vi "运维调试_CODCr.vi"() -> ()   [LabVIEW 2016, in "CODCr库.lvlib"]
uses:
  <vilib>/Utility/miscctls.llb/LVPointTypeDef.ctl
  <vilib>/ptbypt/NI_PtbyPt.lvlib
  <vilib>/Utility/config.llb/NI_LVConfig.lvlib
panel:
  out "数据时间":timestamp format="%<%Y/%m/%d %H:%M:%S>T"
  in  "质控参数":bool
  in  "仪器参数":bool
  in  "MB通信方式选择":enum16{"串口", "TCP"}(ring)
  in  "释放串口":bool
  in  "打开串口":bool
  in  "加标回收测试":bool
  in  "平行样测试":bool
  in  "定时启动":bool
  out "COM口":string
  in  "空白测试":bool
  in  "隐藏按钮":bool
  in  "写入消解温度时长":bool
  in  "保存KB值":bool
  in  "标样核查":bool
  out "启动时间":timestamp format="%<%Y/%m/%d %H:%M:%S>T"
  out "主循环次数":i32
  out "status":bool
  out "启动测量模式":T1(ring)
  out "曲线截距B":sgl format="%#_10g"
  out "曲线斜率K":sgl format="%#_10g"
  out "量程上限":sgl
  out "量程下限":sgl
  out "消解时长":u16
  out "消解温度":u16
  out "测量精度":u16
  out "测量结果":sgl
  out "标样参考值":sgl
  out "量程":u16
  out "工作状态":T1(ring)
  out "仪器时间":timestamp format="%<%X\n%x>T"
  out "关键参数区":T2
  out "状态告警区":T3 {"告警代码" items=["无告警", "缺试剂告警", "缺水样告警", "缺蒸馏水告警", "缺标液告警", "仪表漏液告警", "标定异常告警", "超量程告警", "加热异常", "低试剂预警", "超上限告警", "超下限告警", "仪表内部其他异常", "滴定异常告警", "电极异常告警", "量程切换告警", "参数设置告警", "PH电极电位异常", "电导率电极异常", "浊度光度异常", "溶解氧电极异常", "溶解氧光强异常", "温度异常告警", "PH异常告警", "溶解氧异常告警", "电导率异常告警", "浊度异常告警", "叶绿素异常告警", "藻密度异常告警", "蓝绿藻异常告警", "ORP异常告警", "氨氮异常告警", "清洁刷异常告警", "SD卡异常告警", "蓝牙异常告警", "Wifi异常告警", "流程异常告警"]; "故障代码" items=["无故障", "电机故障", "温度故障", "通讯故障", "滴定故障"]}
  out "测量数据区":T4 {"单位" items=["ug/L", "mg/L", "ppm", "mg/m3", "cm", "ppb", "ug/m3", "%", "nmol/mol", "umol/mol", "MPN/L", "MPN/100ml", "ng/m3", "NTU", "无量纲", "ms/cm", "us/cm", "℃", "mV", "万个/L"]}
  out "系统时间":timestamp format="%<%Y/%m/%d %H:%M:%S>T"
  in  "停止":bool
  in  "校时":bool
  in  "标样校准":bool
  in  "空白校准":bool
  in  "零点核查":bool
  in  "跨度核查":bool
  in  "水样测试":bool
  in  "返回":bool
  in  "设置":bool
  # "mg/L"
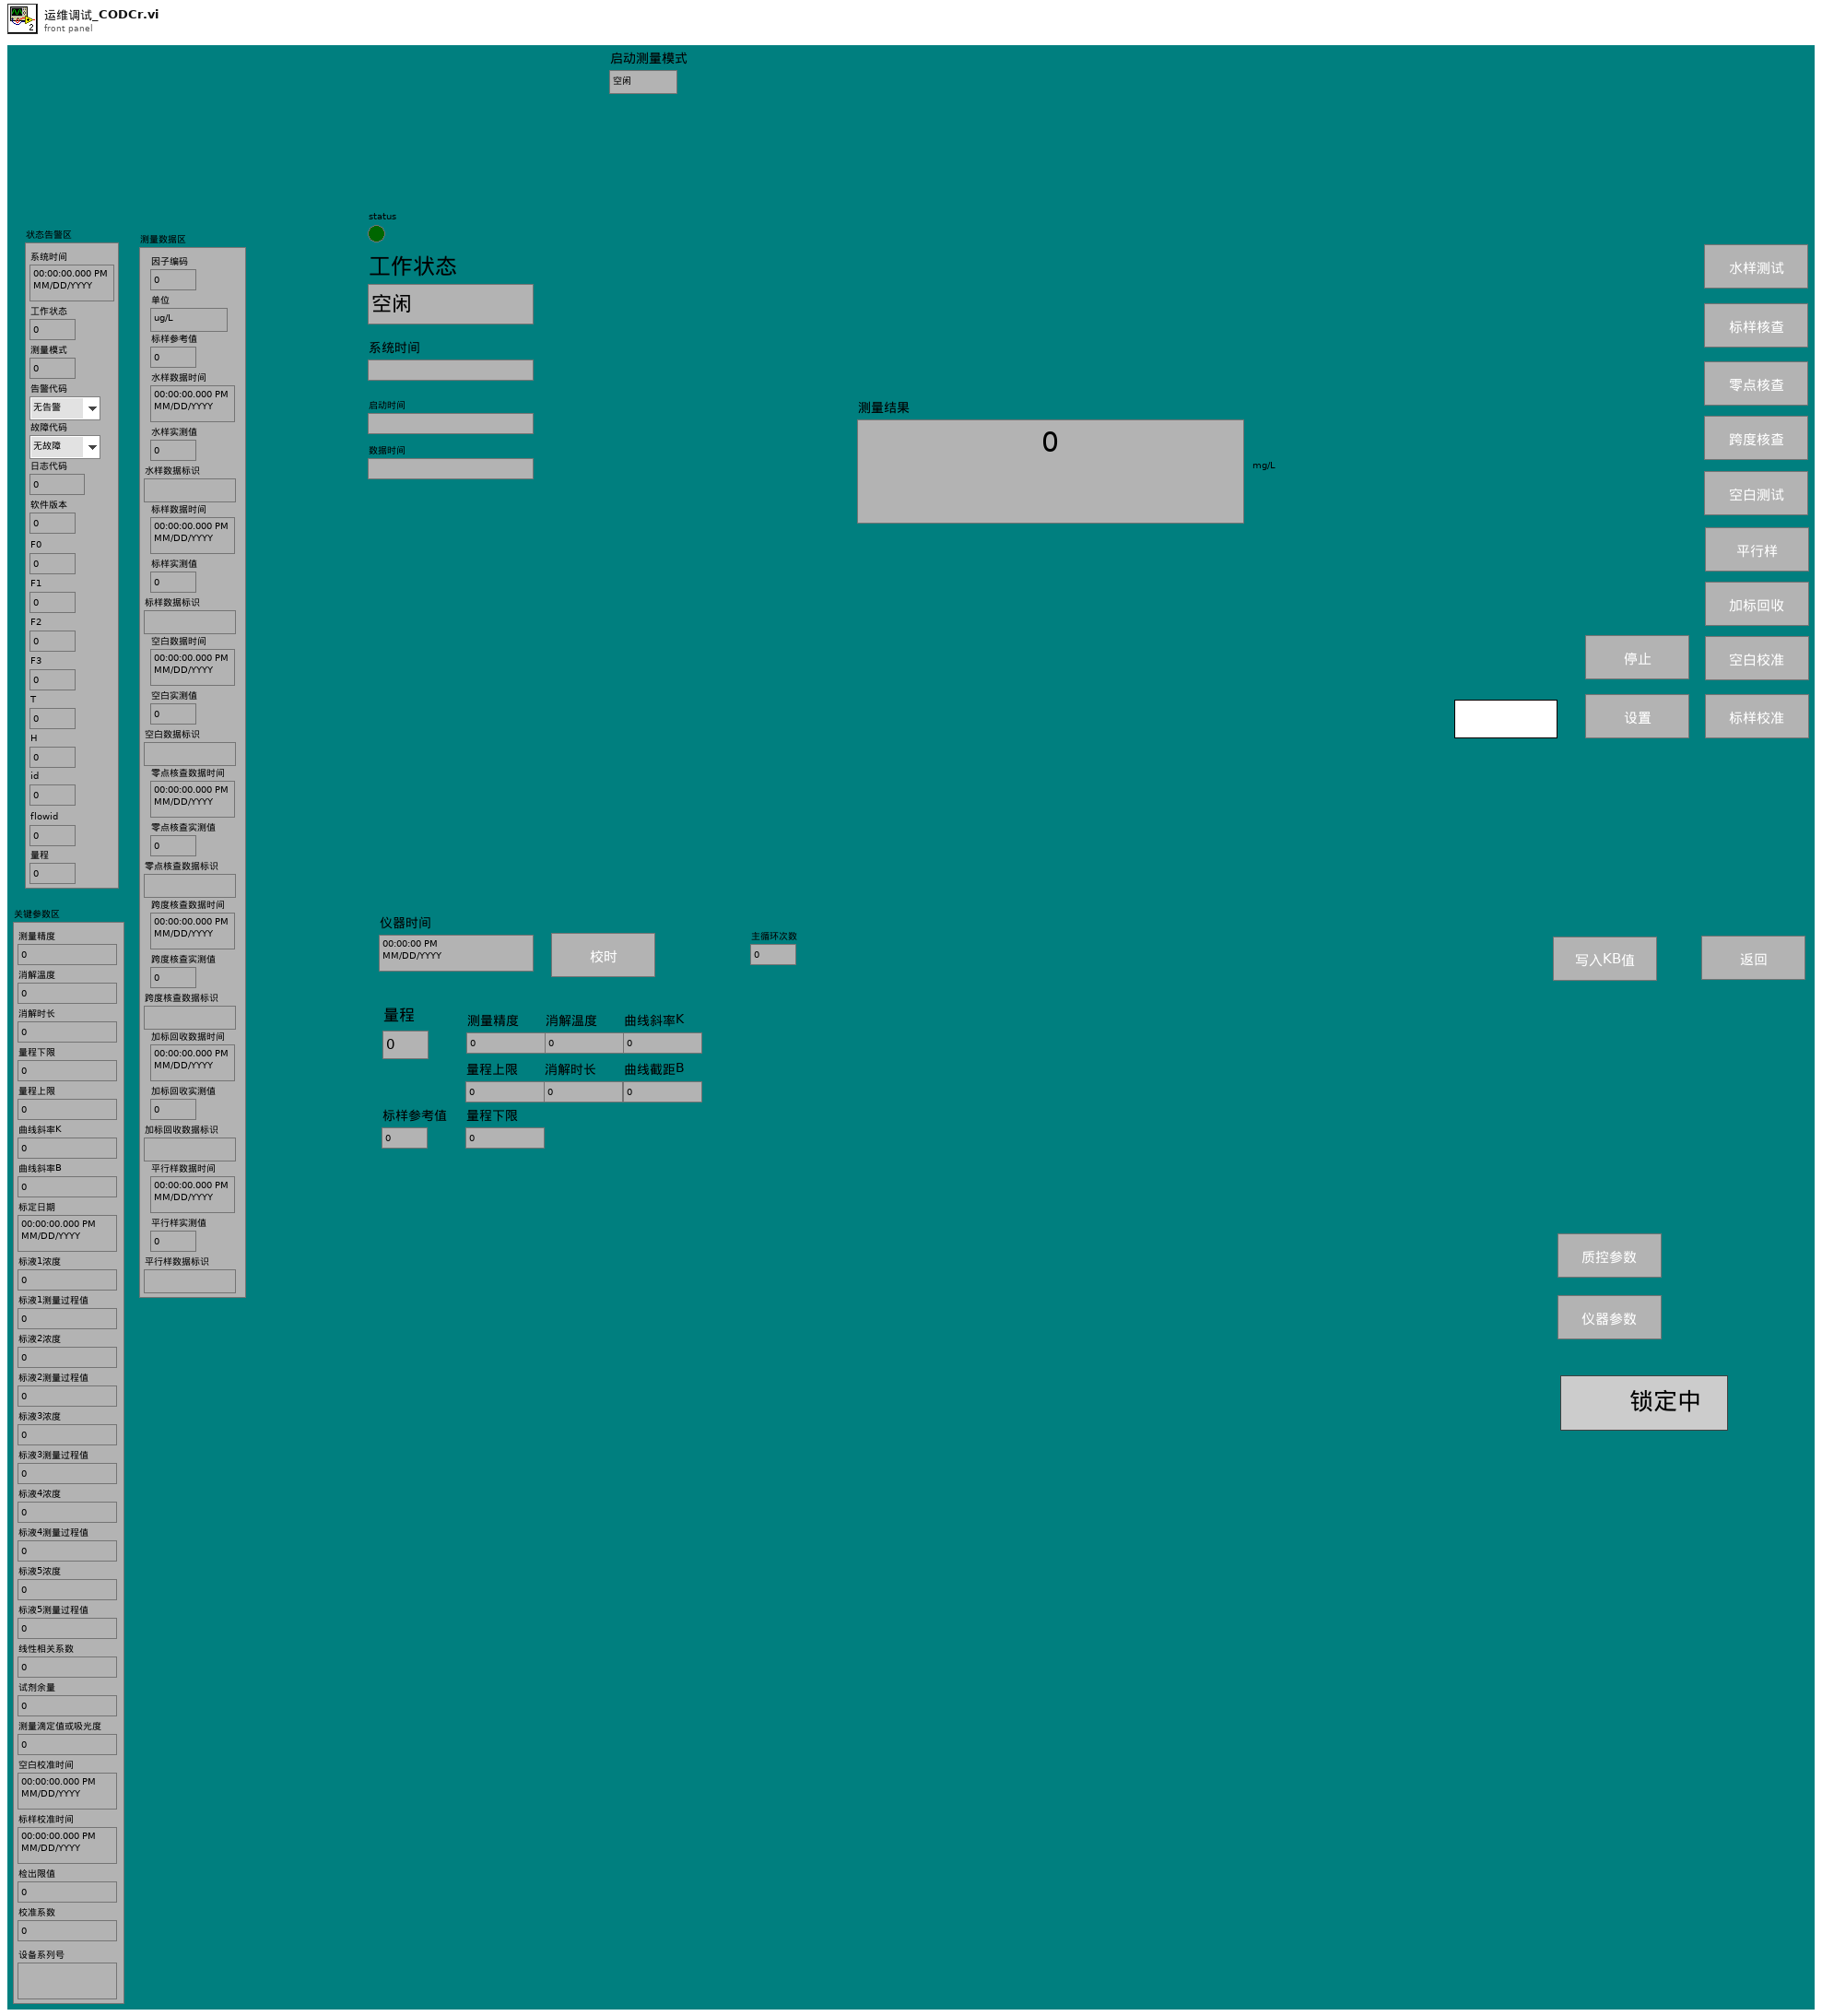
[diagram p1: front panel]
types:
  T1 = enum16{"空闲", "水样测试", "标样核查", "零点核查", "跨度核查", "空白测试", "平行样测试", "加标回收", "空白校准", "标样校准", "初始化（清洗）"}
  T2 = cluster{"测量精度":u16, "消解温度":u16, "消解时长":u16, "量程下限":sgl, "量程上限":sgl, "曲线斜率K":sgl, "曲线斜率B":sgl, "标定日期":timestamp, "标液1浓度":sgl, "标液1测量过程值":sgl, "标液2浓度":sgl, "标液2测量过程值":sgl, "标液3浓度":sgl, "标液3测量过程值":sgl, "标液4浓度":sgl, "标液4测量过程值":sgl, "标液5浓度":sgl, "标液5测量过程值":sgl, "线性相关系数":sgl, "试剂余量":u32, "测量滴定值或吸光度":sgl, "空白校准时间":timestamp, "标样校准时间":timestamp, "检出限值":sgl, "校准系数":sgl, "设备系列号":string}
  T3 = cluster{"系统时间":timestamp, "工作状态":u16, "测量模式":u16, "告警代码":u16, "故障代码":u16, "日志代码":u16, "软件版本":u16, "F0":sgl, "F1":sgl, "F2":sgl, "F3":sgl, "T":sgl, "H":sgl, "id":u16, "flowid":u16, "量程":u16}
  T4 = cluster{"因子编码":u32, "单位":u16, "标样参考值":sgl, "水样数据时间":timestamp, "水样实测值":sgl, "水样数据标识":string, "标样数据时间":timestamp, "标样实测值":sgl, "标样数据标识":string, "空白数据时间":timestamp, "空白实测值":sgl, "空白数据标识":string, "零点核查数据时间":timestamp, "零点核查实测值":sgl, "零点核查数据标识":string, "跨度核查数据时间":timestamp, "跨度核查实测值":sgl, "跨度核查数据标识":string, "加标回收数据时间":timestamp, "加标回收实测值":sgl, "加标回收数据标识":string, "平行样数据时间":timestamp, "平行样实测值":sgl, "平行样数据标识":string}
  T5 = cluster{"命令":string, "测量模式":enum16{"水样测量", "标样核查", "零点核查", "跨度核查", "空白测试", "加标回收", "平行样", "校零", "校标"}, "CODCr量程切换":enum32{"H", "L", "AUTO"}}
  T6 = typedef "LVPointTypeDef.ctl" = cluster{"Horizontal":i16, "Vertical":i16}
  T7 = typedef "NI_LVConfig.lvlib/Config Data RefNum.ctl" = refnum<k1>
  T8 = cluster{"运行模式":enum16{"维护模式", "常规模式", "应急模式", "质控模式"}}
  T9 = cluster{"时间标识":timestamp, "监测值":sgl, "单位":u16, "数据标识":string, "因子编码":u32, "标样参考值":sgl, "F0":sgl, "F1":sgl, "F2":sgl, "F3":sgl, "温度":sgl, "湿度":sgl, "量程标识":string, "LastTime":timestamp}
  T10 = cluster{"时间标识":timestamp, "设备":string, "日志信息":string}
  T11 = cluster{"时间标识":timestamp, "参数":string, "日志信息":string, "流程参数":string}
  T12 = cluster{"时间标识":timestamp, "设备":string, "日志信息":string, "流程参数":string}
  T13 = enum16{"水样测量", "标样核查", "零点核查", "跨度核查", "空白测试", "加标回收", "平行样", "校零", "校标"}
  T14 = cluster{"控制命令":enum16{"启动测量", "标样核查", "零点核查", "跨度核查", "空白测试", "平行样测试", "加标回收", "空白校准", "标样校准", "初始化（清洗）", "停止测试", "仪器重启", "校时", "模式设置", "测量间隔设置"}, "周期设置类型":enum16{"定点启动", "间隔启动"}, "定时功能启用":bool, "定时间隔":dbl, "24H周期设置":bool[], "零点核查时间":u16, "跨度核查时间":u16, "质控频次":enum16{"关闭", "每天", "星期一", "星期二", "星期三", "星期四", "星期五", "星期六", "星期日"}}
  T15 = cluster{"测量量程":dbl, "测量精度":dbl, "测量间隔":dbl, "消解温度":dbl, "消解时长":dbl, "空白校准时间":timestamp, "曲线截距":dbl, "曲线斜率":dbl, "测量检出限":dbl, "测量信号值":dbl, "线性相关系数":dbl, "二次多项式系数":dbl, "标样校准时间":timestamp, "稀释倍数":dbl, "三项式系数":dbl, "空白标定系数":dbl, "量程系数":dbl, "F0/ORPA":dbl, "F1/ORPB":dbl, "F2/ORPK":dbl, "F3":dbl, "F4":dbl, "F5":dbl, "F6":dbl, "F7":dbl, "X0/滴定数":dbl, "量程":dbl}
  T16 = cluster{"控制命令":enum16{"启动测量", "标样核查", "零点核查", "跨度核查", "空白测试", "平行样测试", "加标回收", "空白校准", "标样校准", "初始化（清洗）", "停止测试", "仪器重启", "校时", "模式设置", "测量间隔设置"}, "周期设置类型":enum16{"定点启动", "间隔启动"}, "定时功能启用":bool, "定时间隔":dbl, "24H周期设置":bool[], "空白核查时间":u16, "跨度核查时间":u16, "质控频次":enum16{"关闭", "每天", "星期一", "星期二", "星期三", "星期四", "星期五", "星期六", "星期日"}}
  T17 = cluster{"确定":bool, "测量量程":dbl, "测量精度":dbl, "测量间隔":dbl, "消解温度":dbl, "消解时长":dbl, "空白校准时间":timestamp, "曲线截距":dbl, "曲线斜率":dbl, "测量检出限":dbl, "测量信号值":dbl, "线性相关系数":dbl, "二次多项式系数":dbl, "标样校准时间":timestamp, "稀释倍数":dbl, "三项式系数":dbl, "空白标定系数":dbl, "量程系数":dbl, "F0/ORPA":dbl, "F1/ORPB":dbl, "F2/ORPK":dbl, "F3":dbl, "F4":dbl, "F5":dbl, "F6":dbl, "F7":dbl, "X0/滴定数":dbl, "量程":dbl}
  T18 = cluster{"跨度值":dbl, "零点标准液浓度":dbl, "跨度标准液浓度":dbl, "标准液标准浓度":dbl}
  T19 = cluster{"确定":bool, "跨度值":dbl, "零点标准液浓度":dbl, "跨度标准液浓度":dbl, "标准液标准浓度":dbl}
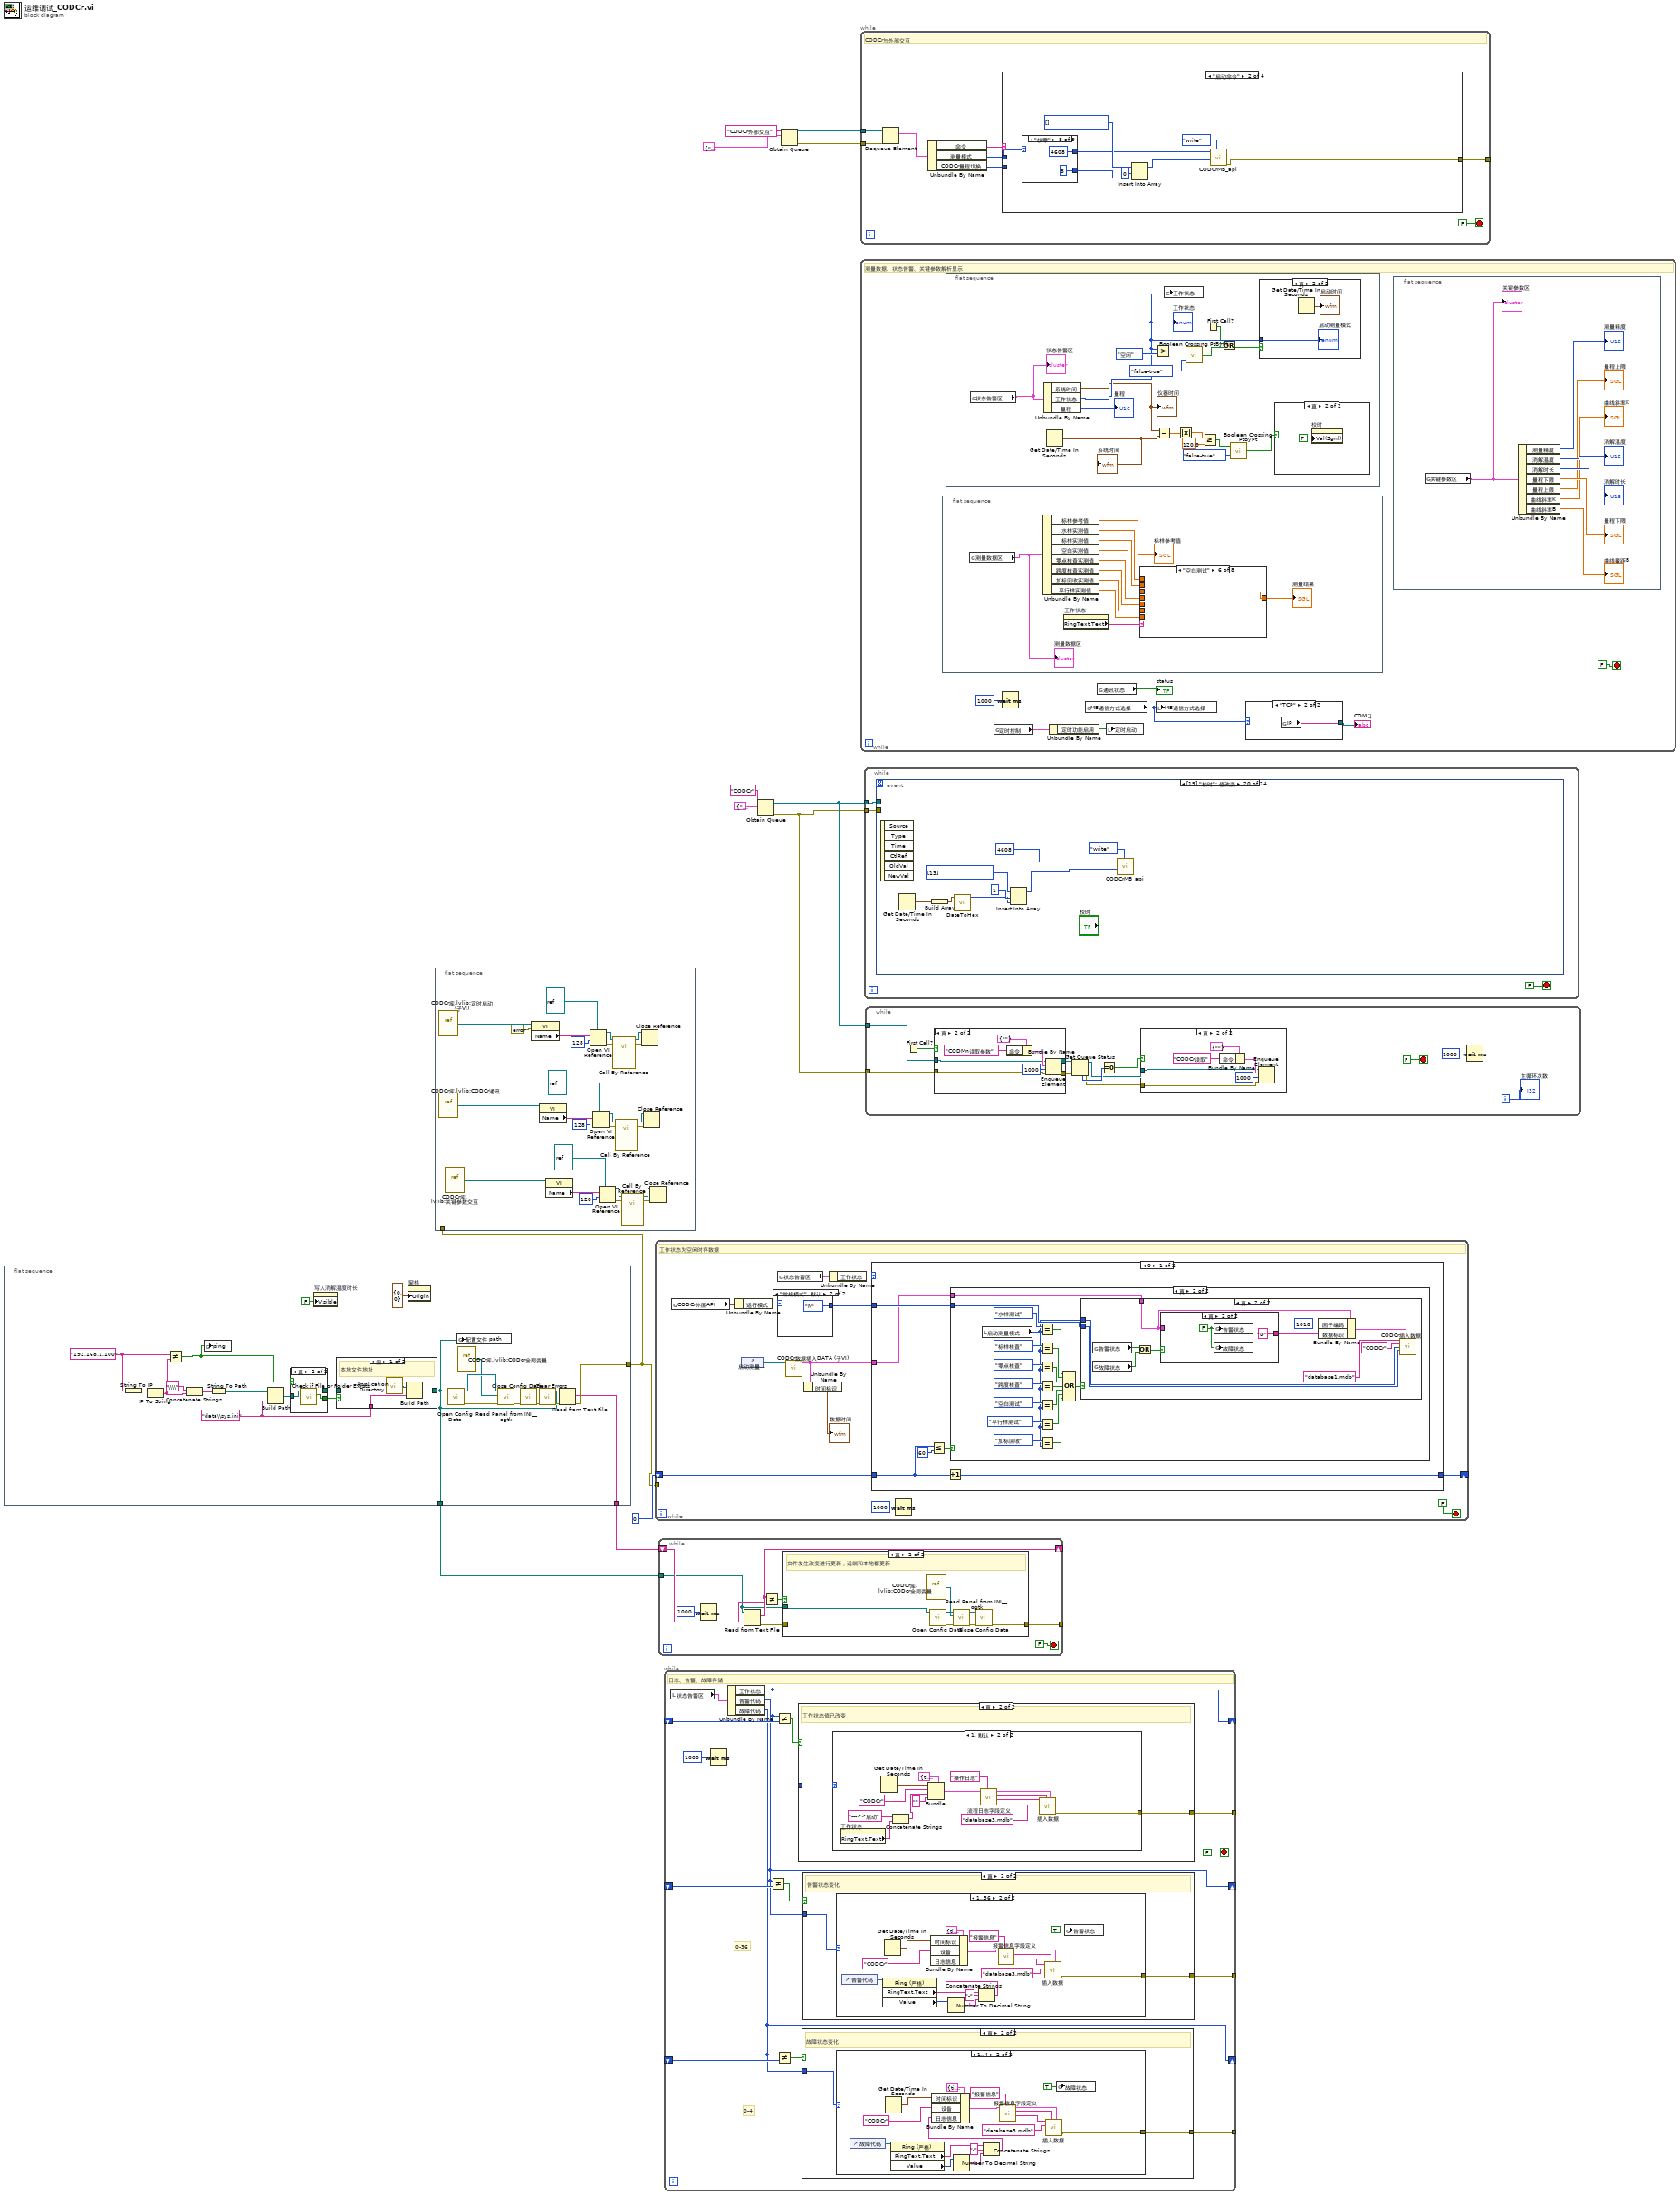
[diagram p0: block diagram]
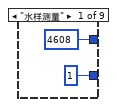
[diagram p6: hidden frame]
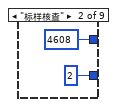
[diagram p7: hidden frame]
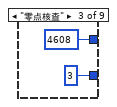
[diagram p8: hidden frame]
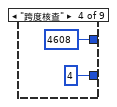
[diagram p9: hidden frame]
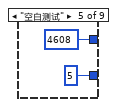
[diagram p10: hidden frame]
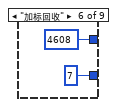
[diagram p11: hidden frame]
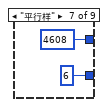
[diagram p12: hidden frame]
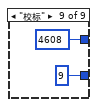
[diagram p13: hidden frame]
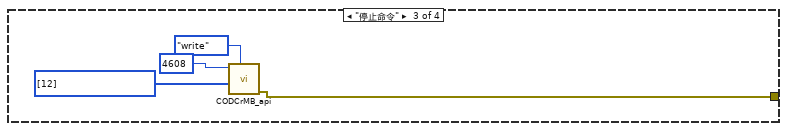
[diagram p14: hidden frame]
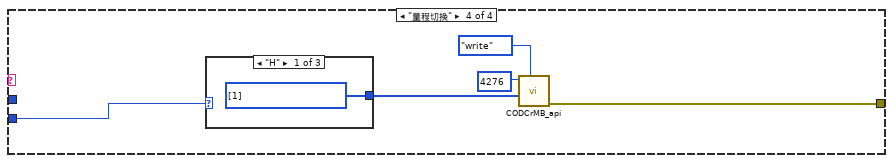
[diagram p15: hidden frame]
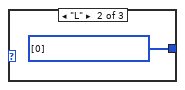
[diagram p16: hidden frame]
diagram:
  n1 = flat-sequence {
    tunnel: [w15] -> w1
    tunnel: [w14] -> w3
    tunnel: [w13] -> w2
    frame #0 {
      w33 = "data\\sys.ini" ("名称或相对路径")
      w18 = "192.168.1.100" ("名称")
      n2 = String To IP(1:w18) -> (0:w25:u32)
      n3 = IP To String(2:w25) -> (0:w22:string)  [unwired: 1 in]
      n4 = Not Equal?(x=w18, y=w22) -> (x != y?=w32:bool)
      n5 = Concatenate Strings("\\\\" ("字符串"), w22) -> (w23:string)
      n6 = global write "CODcr全局变量.vi" "ping"(w32) -> ()
      n7 = String To Path(string=w23) -> (path=w17:path)
      n8 = Build Path(base path=w17, name or relative path=w33) -> (appended path=w21:path)
      n9 = case shown="真" w32 {
        tunnel: w21 -> [w36 w40]
        tunnel: [w36 w39] -> w20
        tunnel: [FALSE w38] -> w19
        frame False {
        }
        frame True {
          n10 = call <vilib>:"Check if File or Folder Exists.vi"("path"=w40) -> ("file or folder exists?"=w38:bool, "dup path"=w39:path)  [unwired: 8 in, 1 out]
        }
      }
      n11 = property on="写入消解温度时长" class="Bool"("Visible"=FALSE ("可见")) -> ()  [unwired: 2 in, 2 out]
      n12 = case shown="假" w19 {
        tunnel: w20 -> [_ w44]
        tunnel: [w42 w44] -> w13
        tunnel: w33 -> [w41 _]
        frame False {
          # "本地文件地址"
          n13 = call <vilib>:"Application Directory.vi"() -> ("Application Directory"=w43:path)
          n14 = Build Path(base path=w43, name or relative path=w41) -> (appended path=w42:path)
        }
        frame True {
          # "网络共享地址"
        }
      }
      n15 = property on="窗格" class="Pane"("Origin"=T6 {"Horizontal"=0, "Vertical"=0} ("原点")) -> ()  [unwired: 2 in, 2 out]
      n16 = call <vilib>:"Open Config Data.vi"("configuration file path"=w13) -> ("error out"=w29:errorcluster, "refnum"=w28:T7)  [unwired: 8 in, 1 out]
      n17 = global write "CODcr全局变量.vi" "配置文件 path"(w13) -> ()
      n18 = vi-ref "CODCr库.lvlib:CODcr全局变量.vi"() -> (w16:refnum<vi>)
      n19 = call <userlib>:"Read Panel from INI__ogtk.vi"("error in (no error)"=w29, "VI ref"=w16, "refnum"=w28) -> ("error out"=w27:errorcluster, "refnum out"=w26:T7)  [unwired: 7 in]
      n20 = call <vilib>:"Close Config Data.vi"("error in (no error)"=w27, "refnum"=w26) -> ("error out"=w30:errorcluster)  [unwired: 8 in, 1 out]
      n21 = call <vilib>:"Clear Errors.vi"("error in (no error)"=w30) -> ("error out"=w31:errorcluster)  [unwired: 5 in, 1 out]
      n22 = Read from Text File(file (use dialog)=w13, error in=w31) -> (text=w14:string, error out=w15:errorcluster)  [unwired: 2 in, 2 out]
    }
  }
  n23 = flat-sequence {
    tunnel: w1 -> [_]
    frame #0 {
      n24 = vi-ref "CODCr库.lvlib:定时启动 (子VI).vi"() -> (w53:refnum<vi>)
      n25 = vi-ref "CODCr库.lvlib:CODCr通讯.vi"() -> (w62:refnum<vi>)
      n26 = vi-ref "CODCr库.lvlib:关键参数交互.vi"() -> (w52:refnum<vi>)
      n27 = property class="VI"(reference=w53, error in=errorcluster {"status"=FALSE, "code"=0, "source"=""} ("错误输出")) -> ("Name"=w54:string)  [unwired: 2 out]
      n28 = property class="VI"(reference=w62) -> ("Name"=w63:string)  [unwired: 1 in, 2 out]
      n29 = property class="VI"(reference=w52) -> ("Name"=w51:string)  [unwired: 1 in, 2 out]
      n30 = Open VI Reference(type specifier VI Refnum (for type only)=refnum<vi> refnum, vi path=w54, options=128 ("选项")) -> (vi reference=w56:refnum<vi>, error out=w58:errorcluster)  [unwired: 3 in]
      n31 = Open VI Reference(type specifier VI Refnum (for type only)=refnum<vi> refnum, vi path=w63, options=128 ("选项")) -> (vi reference=w65:refnum<vi>, error out=w67:errorcluster)  [unwired: 3 in]
      n32 = Open VI Reference(type specifier VI Refnum (for type only)=refnum<vi> refnum, vi path=w51, options=128 ("选项")) -> (vi reference=w49:refnum<vi>, error out=w47:errorcluster)  [unwired: 3 in]
      n33 = call-by-ref "?"(reference=w56, error in=w58) -> (reference out=w60:refnum<vi>, error out=w59:errorcluster)  [unwired: 12 in]
      n34 = call-by-ref "?"(reference=w65, error in=w67) -> (reference out=w69:refnum<vi>, error out=w68:errorcluster)  [unwired: 12 in]
      n35 = call-by-ref "?"(reference=w49, error in=w47) -> (reference out=w45:refnum<vi>, error out=w46:errorcluster)  [unwired: 12 in]
      n36 = Close Reference(reference=w60, error in (no error)=w59) -> ()  [unwired: 1 out]
      n37 = Close Reference(reference=w69, error in (no error)=w68) -> ()  [unwired: 1 out]
      n38 = Close Reference(reference=w45, error in (no error)=w46) -> ()  [unwired: 1 out]
    }
  }
  n39 = while "While循环" {
    tunnel: w1 -> [_]
    shift-right: [w73] -> _
    shift-left: 0 -> [w74]
    stop <- FALSE stop-if-true
    # "工作状态为空闲时存数据"
    n40 = global read "CODCr外部API.vi" "CODCr外围API"() -> (w77:T8)
    n41 = Unbundle By Name(w77) -> ("运行模式"=w76:enum16{"维护模式", "常规模式", "应急模式", "质控模式"})
    n42 = control-ref of="启动测量模式"() -> (w72:refnum<vi>)
    n43 = global read "CODcr全局变量.vi" "状态告警区"() -> (w75:T3)
    n44 = case shown="\"常规模式\", 默认" w76 {
      tunnel: [enum16{"N", "M"}."M" ("数据类型") enum16{"N", "M"}."N" ("数据类型")] -> w78
      frame "维护模式" {
      }
      frame "常规模式", Default {
      }
    }
    n45 = call "CODCr数据插入DATA (子VI).vi"("Enum输入"=w72) -> ("data"=w71:T9)  [unwired: 10 in]
    n46 = Unbundle By Name(w71) -> ("时间标识"=→"数据时间":timestamp)
    n47 = Unbundle By Name(w75) -> ("工作状态"=w79:u16)
    n48 = case shown="0" w79 {
      tunnel: w78 -> [w89 _]
      tunnel: w74 -> [w87 _]
      tunnel: [w88 _] -> w73
      tunnel: w71 -> [w84 _]
      frame 0 {
        n49 = Less Or Equal?(x=w87, y=60) -> (x <= y?=w85:bool)
        n50 = Increment(x=w87) -> (x+1=w88:i32)
        n51 = case shown="真" w85 {
          tunnel: w89 -> [_ w107]
          tunnel: w84 -> [_ w90]
          frame False {
          }
          frame True {
            n52 = local read "启动测量模式"() -> (w99:T1)
            n53 = Equal?(x=T1."水样测试" ("启动测量模式"), y=w99) -> (x = y?=w98:bool)
            n54 = Equal?(x=T1."标样核查" ("启动测量模式"), y=w99) -> (x = y?=w97:bool)
            n55 = Equal?(x=T1."零点核查" ("启动测量模式"), y=w99) -> (x = y?=w96:bool)
            n56 = Equal?(x=T1."跨度核查" ("启动测量模式"), y=w99) -> (x = y?=w95:bool)
            n57 = Equal?(x=T1."空白测试" ("启动测量模式"), y=w99) -> (x = y?=w94:bool)
            n58 = Equal?(x=T1."平行样测试" ("启动测量模式"), y=w99) -> (x = y?=w93:bool)
            n59 = Equal?(x=T1."加标回收" ("启动测量模式"), y=w99) -> (x = y?=w92:bool)
            n60 = Compound Arithmetic op=OR(w98, w97, w96, w95, w94, w93, w92) -> (w91:bool)
            n61 = case shown="真" w91 {
              tunnel: w99 -> [_ w115]
              tunnel: w107 -> [_ w114]
              tunnel: w90 -> [_ w108]
              frame False {
              }
              frame True {
                n62 = global read "CODcr全局变量.vi" "告警状态"() -> (w112:bool)
                n63 = global read "CODcr全局变量.vi" "故障状态"() -> (w111:bool)
                n64 = Or(x=w112, y=w111) -> (x .or. y?=w110:bool)
                n65 = case shown="真" w110 {
                  tunnel: w108 -> [w120 _]
                  tunnel: [w119 "D" ("table")] -> w109
                  frame False {
                    n66 = Unbundle By Name(w120) -> ("数据标识"=w119:string)
                  }
                  frame True {
                    w121 = FALSE ("告警状态")
                    n67 = global write "CODcr全局变量.vi" "告警状态"(w121) -> ()
                    n68 = global write "CODcr全局变量.vi" "故障状态"(w121) -> ()
                  }
                }
                n69 = Bundle By Name(cluster=w108, "因子编码"=u32 1018, "数据标识"=w109) -> (w118:T9)
                n70 = call "CODCr插入数据.vi"("database"="database1.mdb", "data"=w118, "table"="CODCr", "测量模式"=w115, "数据类型"=w114) -> ()  [unwired: 10 in, 1 out]
              }
            }
          }
        }
      }
      frame 1, Default {
      }
    }
    n71 = Wait (ms)(milliseconds to wait=u32 1000 ("等待时间（毫秒）")) -> ()  [unwired: 1 out]
  }
  n72 = while {
    tunnel: [w129] -> _
    shift-right: [w127] -> _
    shift-left: w3 -> [w126]
    tunnel: w2 -> [w123]
    stop <- FALSE stop-if-true
    n73 = Wait (ms)(milliseconds to wait=u32 1000 ("等待时间（毫秒）")) -> ()  [unwired: 1 out]
    n74 = Read from Text File(file (use dialog)=w123) -> (text=w127:string, error out=w124:errorcluster)  [unwired: 3 in, 2 out]
    n75 = Not Equal?(x=w127, y=w126) -> (x != y?=w125:bool)
    n76 = case shown="真" w125 {
      tunnel: [w131 w138] -> w129
      tunnel: w123 -> [_ w132]
      tunnel: w124 -> [w131 _]
      frame False {
      }
      frame True {
        # "文件发生改变进行更新，远端和本地都更新"
        n77 = vi-ref "CODCr库.lvlib:CODcr全局变量.vi"() -> (w133:refnum<vi>)
        n78 = call <vilib>:"Open Config Data.vi"("configuration file path"=w132) -> ("error out"=w137:errorcluster, "refnum"=w136:T7)  [unwired: 8 in, 1 out]
        n79 = call <userlib>:"Read Panel from INI__ogtk.vi"("error in (no error)"=w137, "VI ref"=w133, "refnum"=w136) -> ("error out"=w135:errorcluster, "refnum out"=w134:T7)  [unwired: 7 in]
        n80 = call <vilib>:"Close Config Data.vi"("error in (no error)"=w135, "refnum"=w134) -> ("error out"=w138:errorcluster)  [unwired: 8 in, 1 out]
      }
    }
  }
  n81 = while {
    shift-right: [w149] -> _
    shift-left: _ -> [w151]
    tunnel: [w148] -> _
    shift-right: [w145] -> _
    shift-left: _ -> [w146]
    shift-right: [w141] -> _
    shift-left: _ -> [w143]
    tunnel: [w142] -> _
    tunnel: [w140] -> _
    stop <- FALSE stop-if-true
    # "0-4"
    # "0-36"
    # "日志、告警、故障存储"
    n82 = local read "状态告警区"() -> (w139:T3)
    n83 = Wait (ms)(milliseconds to wait=u32 1000 ("等待时间（毫秒）")) -> ()  [unwired: 1 out]
    n84 = Unbundle By Name(w139) -> ("工作状态"=w149:u16, "告警代码"=w145:u16, "故障代码"=w141:u16)
    n85 = Not Equal?(x=w145, y=w146) -> (x != y?=w147:bool)
    n86 = Not Equal?(x=w149, y=w151) -> (x != y?=w150:bool)
    n87 = Not Equal?(x=w141, y=w143) -> (x != y?=w144:bool)
    n88 = case shown="真" w150 {
      tunnel: w149 -> [_ w193]
      tunnel: [_ w192] -> w148
      frame False {
      }
      frame True {
        # "工作状态值已改变"
        n89 = case shown="1, 默认" w193 {
          tunnel: [w194 w209] -> w192
          frame 0 {
            n90 = Get Date/Time In Seconds() -> (seconds since 1Jan1904=w201:timestamp)
            n91 = Bundle(cluster=T11 {"时间标识"=timestamp(0 s since 1904-01-01), "参数"="", "日志信息"="", "流程参数"=""} ("data in"), "时间标识"=w201, "参数"="CODCr" ("table输入"), "日志信息"="--->>结束", "流程参数"="" ("table输入")) -> (w195:T11)
            n92 = call "流程日志字段定义.vi"("table输入"="操作日志", "data in"=w195) -> ("table输出"=w199:string, "columns"=w197:string[], "data out"=w196:T12)  [unwired: 7 in]
            n93 = call "插入数据.vi"("data"=w196, "columns"=w197, "database"="database3.mdb", "table"=w199) -> ("error out"=w194:errorcluster)  [unwired: 7 in]
          }
          frame 1, Default {
            n94 = property on="工作状态" class="Enum (严格)"() -> ("RingText.Text"=w206:string)  [unwired: 2 in, 2 out]
            n95 = Get Date/Time In Seconds() -> (seconds since 1Jan1904=w216:timestamp)
            n96 = Concatenate Strings("--->>启动" ("日志信息"), w206) -> (w207:string)
            n97 = Bundle(cluster=T11 {"时间标识"=timestamp(0 s since 1904-01-01), "参数"="", "日志信息"="", "流程参数"=""} ("data in"), "时间标识"=w216, "参数"="CODCr" ("table输入"), "日志信息"=w207, "流程参数"="" ("table输入")) -> (w215:T11)
            n98 = call "流程日志字段定义.vi"("table输入"="操作日志", "data in"=w215) -> ("table输出"=w213:string, "columns"=w211:string[], "data out"=w210:T12)  [unwired: 7 in]
            n99 = call "插入数据.vi"("data"=w210, "columns"=w211, "database"="database3.mdb", "table"=w213) -> ("error out"=w209:errorcluster)  [unwired: 7 in]
          }
        }
      }
    }
    n100 = case shown="真" w144 {
      tunnel: w141 -> [_ w155]
      tunnel: [_ w154] -> w140
      frame False {
      }
      frame True {
        # "故障状态变化"
        n101 = case shown="1..4" w155 {
          tunnel: [_ w162] -> w154
          frame 0, Default {
            # "无告警"
          }
          frame 1..4 {
            n102 = control-ref of="故障代码"() -> (w172:refnum<vi>)
            n103 = Get Date/Time In Seconds() -> (seconds since 1Jan1904=w170:timestamp)
            n104 = property class="Ring (严格)"(reference=w172) -> ("RingText.Text"=w159:string, "Value"=w160:u16)  [unwired: 1 in, 2 out]
            n105 = Number To Decimal String(number=w160) -> (decimal integer string=w157:string)  [unwired: 1 in]
            n106 = Concatenate Strings(w159, "-" ("字符串"), w157) -> (w158:string)
            n107 = Bundle By Name(cluster=T10 {"时间标识"=timestamp(0 s since 1904-01-01), "设备"="", "日志信息"=""} ("data in"), "时间标识"=w170, "设备"="CODCr" ("table输入"), "日志信息"=w158) -> (w169:T10)
            n108 = call "报警信息字段定义.vi"("table输入"="报警信息", "data in"=w169) -> ("table输出"=w164:string, "columns"=w163:string[], "data out"=w166:T10)  [unwired: 7 in]
            n109 = call "插入数据.vi"("data"=w166, "columns"=w163, "database"="database3.mdb", "table"=w164) -> ("error out"=w162:errorcluster)  [unwired: 7 in]
            n110 = global write "CODcr全局变量.vi" "故障状态"(TRUE ("告警状态")) -> ()
          }
        }
      }
    }
    n111 = case shown="真" w147 {
      tunnel: w145 -> [_ w174]
      tunnel: [_ w173] -> w142
      frame False {
      }
      frame True {
        # "告警状态变化"
        n112 = case shown="1..36" w174 {
          tunnel: [_ w184] -> w173
          frame 0, Default {
            # "无告警"
          }
          frame 1..36 {
            n113 = control-ref of="告警代码"() -> (w181:refnum<vi>)
            n114 = property class="Ring (严格)"(reference=w181) -> ("RingText.Text"=w179:string, "Value"=w178:u16)  [unwired: 1 in, 2 out]
            n115 = Get Date/Time In Seconds() -> (seconds since 1Jan1904=w183:timestamp)
            n116 = Number To Decimal String(number=w178) -> (decimal integer string=w175:string)  [unwired: 1 in]
            n117 = Concatenate Strings(w179, "-" ("字符串"), w175) -> (w177:string)
            n118 = Bundle By Name(cluster=T10 {"时间标识"=timestamp(0 s since 1904-01-01), "设备"="", "日志信息"=""} ("data in"), "时间标识"=w183, "设备"="CODCr" ("table输入"), "日志信息"=w177) -> (w185:T10)
            n119 = call "报警信息字段定义.vi"("table输入"="报警信息", "data in"=w185) -> ("table输出"=w190:string, "columns"=w191:string[], "data out"=w188:T10)  [unwired: 7 in]
            n120 = call "插入数据.vi"("data"=w188, "columns"=w191, "database"="database3.mdb", "table"=w190) -> ("error out"=w184:errorcluster)  [unwired: 7 in]
            n121 = global write "CODcr全局变量.vi" "告警状态"(TRUE ("告警状态")) -> ()
          }
        }
      }
    }
  }
  n122 = Obtain Queue(name (unnamed)="CODCr" ("名称（未命名）"), element data type=cluster{"命令":string} {"命令"="启用模块"} ("元素")) -> (queue out=w6:refnum<queue>, error out=w5:errorcluster)  [unwired: 3 in, 1 out]
  n123 = Obtain Queue(name (unnamed)="CODCr外部交互" ("名称（未命名）"), element data type=T5 {"命令"="启动命令", "测量模式"=enum."水样测量", "CODCr量程切换"=enum."AUTO"} ("元素")) -> (queue out=w8:refnum<queue>, error out=w7:errorcluster)  [unwired: 3 in, 1 out]
  n124 = while {
    tunnel: w8 -> [w225]
    tunnel: w7 -> [w224]
    tunnel: [w220] -> _
    stop <- FALSE stop-if-true
    # "CODCr与外部交互"
    n125 = Dequeue Element(queue=w225, error in (no error)=w224) -> (element=w226:T5)  [unwired: 1 in, 3 out]
    n126 = Unbundle By Name(w226) -> ("命令"=w223:string, "测量模式"=w222:T13, "CODCr量程切换"=w221:enum32{"H", "L", "AUTO"})
    n127 = case shown="\"启动命令\"" w223 {
      tunnel: w222 -> [_ w229 _ _]
      tunnel: w221 -> [_ _ _ w259]
      tunnel: [_ w228 w254 w258] -> w220
      frame "假", Default {
      }
      frame "启动命令" {
        n128 = case shown="\"校零\"" w229 {
          tunnel: [u16 4608 ("address") u16 4608 ("address") u16 4608 ("address") u16 4608 ("address") u16 4608 ("address") u16 4608 ("address") u16 4608 ("address") u16 4608 ("address") u16 4608 ("address")] -> w231
          tunnel: [u16 1 ("address") u16 2 ("address") u16 3 ("address") u16 4 ("address") u16 5 ("address") u16 7 ("address") u16 6 ("address") u16 8 ("address") u16 9 ("address")] -> w235
          frame "水样测量" {
          }
          frame "标样核查" {
          }
          frame "零点核查" {
          }
          frame "跨度核查" {
          }
          frame "空白测试" {
          }
          frame "加标回收" {
          }
          frame "平行样" {
          }
          frame "校零" {
          }
          frame "校标" {
          }
        }
        n129 = Insert Into Array(array=u16[] [] ("values"), index=0 ("索引"), new element=w235) -> (w230:u16[])
        n130 = call "CODCrMB_api.vi"("STEP"=enum16{"open", "read", "write", "close"}."write", "values"=w230, "starting address"=w231) -> ("error out"=w228:errorcluster)  [unwired: 6 in, 2 out]
      }
      frame "停止命令" {
        n131 = call "CODCrMB_api.vi"("STEP"=enum16{"open", "read", "write", "close"}."write", "values"=u16[] [12], "starting address"=u16 4608) -> ("error out"=w254:errorcluster)  [unwired: 6 in, 2 out]
      }
      frame "量程切换" {
        n132 = case shown="\"H\"" w259 {
          tunnel: [u16[] [1] ("values") u16[] [0] ("values") _] -> w262
          frame "H" {
          }
          frame "L" {
          }
          frame "AUTO", Default {
          }
        }
        n133 = call "CODCrMB_api.vi"("STEP"=enum16{"open", "read", "write", "close"}."write", "values"=w262, "starting address"=u16 4276) -> ("error out"=w258:errorcluster)  [unwired: 6 in, 2 out]
      }
    }
  }
  n134 = while {
    stop <- FALSE stop-if-true
    # "测量数据、状态告警、关键参数解析显示"
    n135 = flat-sequence {
      frame #0 {
        n136 = global read "CODcr全局变量.vi" "测量数据区"() -> (w302:T4)
        "测量数据区" <- w302
        n137 = Unbundle By Name(w302) -> ("标样参考值"=→"标样参考值":sgl, "水样实测值"=w310:sgl, "标样实测值"=w308:sgl, "空白实测值"=w305:sgl, "零点核查实测值"=w307:sgl, "跨度核查实测值"=w306:sgl, "加标回收实测值"=w303:sgl, "平行样实测值"=w304:sgl)
        n138 = property on="工作状态" class="Enum (严格)"() -> ("RingText.Text"=w311:string)  [unwired: 2 in, 2 out]
        n139 = case shown="\"空白测试\"" w311 {
          tunnel: w310 -> [_ w314 _ _ _ _ _ _]
          tunnel: [w313 w314 w315 w316 w317 w318 w319 w320] -> w309
          tunnel: w308 -> [_ _ w315 _ _ _ _ _]
          tunnel: w307 -> [_ _ _ w316 _ _ _ _]
          tunnel: w306 -> [_ _ _ _ w317 _ _ _]
          tunnel: w305 -> [_ _ _ _ _ w318 _ _]
          tunnel: w304 -> [_ _ _ _ _ _ w319 _]
          tunnel: w303 -> [_ _ _ _ _ _ _ w320]
          frame "空闲", Default {
            n140 = local read "测量结果"() -> (w313:sgl)
          }
          frame "水样测试" {
          }
          frame "标样核查" {
          }
          frame "零点核查" {
          }
          frame "跨度核查" {
          }
          frame "空白测试" {
          }
          frame "平行样测试" {
          }
          frame "加标回收" {
          }
        }
        "测量结果" <- w309
      }
    }
    n141 = flat-sequence {
      frame #0 {
        n142 = global read "CODcr全局变量.vi" "状态告警区"() -> (w290:T3)
        "状态告警区" <- w290
        n143 = Unbundle By Name(w290) -> ("系统时间"=w289:timestamp, "工作状态"=w293:u16, "量程"=→"量程":u16)
        "仪器时间" <- w289
        "工作状态" <- w293
        n144 = Get Date/Time In Seconds() -> (seconds since 1Jan1904=w288:timestamp)
        "系统时间" <- w288
        n145 = Greater?(x=w293, y=T1."空闲") -> (0:w297:bool)
        n146 = Subtract(x=w289, y=w288) -> (x-y=w287:dbl)
        n147 = global write "CODcr全局变量.vi" "工作状态"(w293) -> ()
        n148 = Absolute Value(x=w287) -> (abs(x)=w286:dbl)
        n149 = call <vilib>:"Boolean Crossing PtByPt.vi"("direction"=enum16{"either", "false-true", "true-false"}."false-true", "input"=w297) -> ("crossing"=w296:bool)  [unwired: 1 in]
        n150 = Greater Or Equal?(x=w286, y=120.0) -> (x >= y?=w284:bool)
        n151 = First Call?() -> (First Call?: T/F=w291:bool)
        n152 = Or(x=w291, y=w296) -> (x .or. y?=w292:bool)
        n153 = call <vilib>:"Boolean Crossing PtByPt.vi"("direction"=enum16{"either", "false-true", "true-false"}."false-true", "input"=w284) -> ("crossing"=w283:bool)  [unwired: 1 in]
        n154 = case shown="真" w292 {
          tunnel: w293 -> [_ w300]
          frame False {
          }
          frame True {
            n155 = Get Date/Time In Seconds() -> (seconds since 1Jan1904=→"启动时间":timestamp)
            "启动测量模式" <- w300
          }
        }
        n156 = case shown="真" w283 {
          frame False {
          }
          frame True {
            n157 = property on="校时" class="Bool (严格)"("Val(Sgnl)"=TRUE ("值(信号)")) -> ()  [unwired: 2 in, 2 out]
          }
        }
      }
    }
    n158 = global read "CODcr全局变量.vi" "定时控制"() -> (w266:T14)
    n159 = Wait (ms)(milliseconds to wait=u32 1000 ("等待时间（毫秒）")) -> ()  [unwired: 1 out]
    n160 = Unbundle By Name(w266) -> ("定时功能启用"=w265:bool)
    n161 = global read "CODcr全局变量.vi" "MB通信方式选择"() -> (w267:enum16{"串口", "TCP"})
    n162 = global read "CODcr全局变量.vi" "通讯状态"() -> (→"status":bool)
    n163 = local write "定时启动"(w265) -> ()
    n164 = local write "MB通信方式选择"(w267) -> ()
    n165 = case shown="\"TCP\"" w267 {
      tunnel: [w272 w273] -> w268
      frame "串口", Default {
        n166 = global read "CODcr全局变量.vi" "VISA Resource"() -> (w272:refnum<visa-resource-name>)
      }
      frame "TCP" {
        n167 = global read "CODcr全局变量.vi" "IP"() -> (w273:string)
      }
    }
    "COM口" <- w268
    n168 = flat-sequence {
      frame #0 {
        n169 = global read "CODcr全局变量.vi" "关键参数区"() -> (w274:T2)
        "关键参数区" <- w274
        n170 = Unbundle By Name(w274) -> ("测量精度"=→"测量精度":u16, "消解温度"=→"消解温度":u16, "消解时长"=→"消解时长":u16, "量程下限"=→"量程下限":sgl, "量程上限"=→"量程上限":sgl, "曲线斜率K"=→"曲线斜率K":sgl, "曲线斜率B"=→"曲线截距B":sgl)
      }
    }
  }
  n171 = while {
    tunnel: w6 -> [w322]
    tunnel: w5 -> [w321]
    stop <- FALSE stop-if-true
    n172 = event shown="[19] \"校时\": 值改变" {
      selector: _ -> [_ _ _ _ _ _ _ _ _ _ _ _ _ _ _ _ _ _ _ _ _ _ _ _]
      dyn-events: _ -> [_ _ _ _ _ _ _ _ _ _ _ _ _ _ _ _ _ _ _ _ _ _ _ _]
      timeout: _ -> [_ _ _ _ _ _ _ _ _ _ _ _ _ _ _ _ _ _ _ _ _ _ _ _]
      tunnel: w322 -> [_ _ _ _ _ _ _ _ _ _ _ _ _ _ _ w422 w441 _ _ _ w465 _ _ _]
      tunnel: w321 -> [_ _ _ _ _ _ _ _ _ _ _ _ _ _ _ w421 w440 _ _ _ w464 _ _ _]
      event Timeout {
        n173 = event-data() -> ()  [unwired: 1 in, 2 out]
      }
      event "水样测试": Value Change {
        n174 = event-data() -> ()  [unwired: 1 in, 6 out]
        n175 = local write "启动测量模式"(T1."水样测试" ("启动测量模式")) -> ()
        n176 = call "CODCrMB_api.vi"("STEP"=enum16{"open", "read", "write", "close"}."write", "values"=u16[] [1], "starting address"=u16 4608) -> ()  [unwired: 6 in, 3 out]
      }
      event "标样核查": Value Change {
        n177 = event-data() -> ()  [unwired: 1 in, 6 out]
        n178 = local write "启动测量模式"(T1."标样核查" ("启动测量模式")) -> ()
        n179 = call "CODCrMB_api.vi"("STEP"=enum16{"open", "read", "write", "close"}."write", "values"=u16[] [2], "starting address"=u16 4608) -> ()  [unwired: 6 in, 3 out]
      }
      event "零点核查": Value Change {
        n180 = event-data() -> ()  [unwired: 1 in, 6 out]
        n181 = local write "启动测量模式"(T1."零点核查" ("启动测量模式")) -> ()
        n182 = call "CODCrMB_api.vi"("STEP"=enum16{"open", "read", "write", "close"}."write", "values"=u16[] [3], "starting address"=u16 4608) -> ()  [unwired: 6 in, 3 out]
      }
      event "跨度核查": Value Change {
        n183 = event-data() -> ()  [unwired: 1 in, 6 out]
        n184 = local write "启动测量模式"(T1."跨度核查" ("启动测量模式")) -> ()
        n185 = call "CODCrMB_api.vi"("STEP"=enum16{"open", "read", "write", "close"}."write", "values"=u16[] [4], "starting address"=u16 4608) -> ()  [unwired: 6 in, 3 out]
      }
      event "空白测试": Value Change {
        n186 = event-data() -> ()  [unwired: 1 in, 6 out]
        n187 = local write "启动测量模式"(T1."空白测试" ("启动测量模式")) -> ()
        n188 = call "CODCrMB_api.vi"("STEP"=enum16{"open", "read", "write", "close"}."write", "values"=u16[] [5], "starting address"=u16 4608) -> ()  [unwired: 6 in, 3 out]
      }
      event "平行样测试": Value Change {
        n189 = event-data() -> ()  [unwired: 1 in, 6 out]
        n190 = local write "启动测量模式"(T1."平行样测试" ("启动测量模式")) -> ()
        n191 = call "CODCrMB_api.vi"("STEP"=enum16{"open", "read", "write", "close"}."write", "values"=u16[] [6], "starting address"=u16 4608) -> ()  [unwired: 6 in, 3 out]
      }
      event "加标回收测试": Value Change {
        n192 = event-data() -> ()  [unwired: 1 in, 6 out]
        n193 = local write "启动测量模式"(T1."加标回收" ("启动测量模式")) -> ()
        n194 = call "CODCrMB_api.vi"("STEP"=enum16{"open", "read", "write", "close"}."write", "values"=u16[] [7], "starting address"=u16 4608) -> ()  [unwired: 6 in, 3 out]
      }
      event "空白校准": Value Change {
        n195 = event-data() -> ()  [unwired: 1 in, 6 out]
        n196 = local write "启动测量模式"(T1."空白校准" ("启动测量模式")) -> ()
        n197 = call "CODCrMB_api.vi"("STEP"=enum16{"open", "read", "write", "close"}."write", "values"=u16[] [8], "starting address"=u16 4608) -> ()  [unwired: 6 in, 3 out]
      }
      event "标样校准": Value Change {
        n198 = event-data() -> ()  [unwired: 1 in, 6 out]
        n199 = local write "启动测量模式"(T1."标样校准" ("启动测量模式")) -> ()
        n200 = call "CODCrMB_api.vi"("STEP"=enum16{"open", "read", "write", "close"}."write", "values"=u16[] [9], "starting address"=u16 4608) -> ()  [unwired: 6 in, 3 out]
      }
      event "停止": Value Change {
        n201 = event-data() -> ()  [unwired: 1 in, 6 out]
        n202 = Two Button Dialog(message="确认是否停止？" ("消息"), 1:"否" ("F按钮名称（“取消”）"), 2:"是" ("T按钮名称（“确定”）")) -> (T button?=w360:bool)
        n203 = case shown="真" w360 {
          frame False {
          }
          frame True {
            n204 = Obtain Notifier(name (unnamed)="CODCr" ("名称（未命名）"), notification data type=FALSE) -> (notifier out=w368:refnum<notifier>, error out=w366:errorcluster)  [unwired: 2 in, 1 out]
            n205 = call "CODCrMB_api.vi"("STEP"=enum16{"open", "read", "write", "close"}."write", "values"=u16[] [12], "starting address"=u16 4608) -> ()  [unwired: 6 in, 3 out]
            n206 = Send Notification(notification=TRUE ("通知"), notifier=w368, error in (no error)=w366) -> (notifier out=w365:refnum<notifier>, error out=w364:errorcluster)
            n207 = Release Notifier(notifier=w365, error in (no error)=w364) -> ()  [unwired: 1 in, 3 out]
          }
        }
      }
      event "保存KB值": Value Change {
        n208 = event-data() -> ()  [unwired: 1 in, 6 out]
        n209 = local read "曲线截距B"() -> (w374:sgl)
        n210 = local read "曲线斜率K"() -> (w375:sgl)
        n211 = Build Array(w375, w374) -> (w380:sgl[])
        n212 = call "FloatToHex.vi"("浮点数"=w380) -> ("DCBA整形输出"=w377:u16[])  [unwired: 10 in]
        n213 = call "CODCrMB_api.vi"("STEP"=enum16{"open", "read", "write", "close"}."write", "values"=w377, "starting address"=u16 4263) -> ("error out"=w376:errorcluster)  [unwired: 6 in, 2 out]
        n214 = case shown="无错误" w376 {
          tunnel: w375 -> [w382 _]
          tunnel: w374 -> [w381 _]
          frame No Error {
            n215 = global read "CODcr全局变量.vi" "CODCr仪器参数"() -> (w384:T15)
            n216 = Bundle By Name(cluster=w384, "曲线截距"=w381, "曲线斜率"=w382) -> (w383:T15)
            n217 = global write "CODcr全局变量.vi" "CODCr仪器参数"(w383) -> ()
          }
          frame Error {
          }
        }
      }
      event "定时启动": Value Change {
        n218 = event-data() -> ()  [unwired: 1 in, 6 out]
        n219 = flat-sequence {
          frame #0 {
            n220 = global read "CODcr全局变量.vi" "定时控制"() -> (w386:T14)
            n221 = call "周期设置.vi"("定时控制输入"=w386) -> ("定时控制输出"=w385:T16)  [unwired: 10 in]
            n222 = global write "CODcr全局变量.vi" "定时控制"(w385) -> ()
          }
          frame #1 {
            n223 = call "配置文件保存.vi"() -> ()  [unwired: 12 in]
          }
        }
      }
      event "仪器参数": Value Change {
        n224 = event-data() -> ()  [unwired: 1 in, 6 out]
        n225 = global read "CODcr全局变量.vi" "CODCr仪器参数"() -> (w388:T15)
        n226 = call "仪器参数设置.vi"("氨氮仪器参数"=w388) -> ("仪器参数设置输出"=w387:T17)  [unwired: 10 in]
        n227 = Unbundle By Name(w387) -> ("确定"=w389:bool)
        n228 = case shown="真" w389 {
          tunnel: w388 -> [_ w391]
          tunnel: w387 -> [_ w390]
          frame False {
          }
          frame True {
            n229 = flat-sequence {
              tunnel: w391 -> [w408]
              tunnel: w390 -> [w407]
              frame #0 {
                n230 = Unbundle By Name(w407) -> ("测量量程"=w406:dbl, "测量精度"=w405:dbl, "测量间隔"=w404:dbl, "消解温度"=w403:dbl, "消解时长"=w402:dbl, "空白校准时间"=w401:timestamp, "曲线截距"=w400:dbl, "曲线斜率"=w399:dbl, "测量检出限"=w398:dbl, "测量信号值"=w397:dbl, "线性相关系数"=w396:dbl, "二次多项式系数"=w395:dbl, "标样校准时间"=w394:timestamp, "稀释倍数"=w393:dbl)
                n231 = Bundle By Name(cluster=w408, "测量量程"=w406, "测量精度"=w405, "测量间隔"=w404, "消解温度"=w403, "消解时长"=w402, "空白校准时间"=w401, "曲线截距"=w400, "曲线斜率"=w399, "测量检出限"=w398, "测量信号值"=w397, "线性相关系数"=w396, "二次多项式系数"=w395, "标样校准时间"=w394, "稀释倍数"=w393) -> (w392:T15)
                n232 = global write "CODcr全局变量.vi" "CODCr仪器参数"(w392) -> ()
              }
              frame #1 {
                n233 = call "配置文件保存.vi"() -> ()  [unwired: 12 in]
              }
            }
          }
        }
      }
      event "质控参数": Value Change {
        n234 = event-data() -> ()  [unwired: 1 in, 6 out]
        n235 = global read "CODcr全局变量.vi" "质控参数设置"() -> (w410:T18)
        n236 = call "质控参数设置.vi"("质控参数设置"=w410) -> ("输出簇"=w409:T19)  [unwired: 10 in]
        n237 = Unbundle By Name(w409) -> ("确定"=w411:bool)
        n238 = case shown="真" w411 {
          tunnel: w410 -> [_ w413]
          tunnel: w409 -> [_ w412]
          frame False {
          }
          frame True {
            n239 = flat-sequence {
              tunnel: w413 -> [w420]
              tunnel: w412 -> [w419]
              frame #0 {
                n240 = Unbundle By Name(w419) -> ("跨度值"=w417:dbl, "零点标准液浓度"=w416:dbl, "跨度标准液浓度"=w415:dbl, "标准液标准浓度"=w414:dbl)
                n241 = Bundle By Name(cluster=w420, "跨度值"=w417, "零点标准液浓度"=w416, "跨度标准液浓度"=w415, "标准液标准浓度"=w414) -> (w418:T18)
                n242 = global write "CODcr全局变量.vi" "质控参数设置"(w418) -> ()
              }
              frame #1 {
                n243 = call "配置文件保存.vi"() -> ()  [unwired: 12 in]
              }
            }
          }
        }
      }
      event "打开串口": Value Change {
        n244 = event-data() -> ()  [unwired: 1 in, 6 out]
        n245 = flat-sequence {
          tunnel: w422 -> [w424]
          tunnel: w421 -> [w423]
          frame #0 {
            n246 = global read "CODcr全局变量.vi" "VISA Resource"() -> (w431:refnum<visa-resource-name>)
            n247 = global read "CODcr全局变量.vi" "PORT"() -> (w425:string)
            n248 = global read "CODcr全局变量.vi" "IP"() -> (w426:string)
            n249 = call "串口配置.vi"("PORT"=w425, "IP"=w426, "请选择串口:"=w431) -> ("PORT 2"=w427:string, "IP 2"=w428:string, "确认 2"=w430:bool, "VISA资源名称 2"=w429:refnum<visa-resource-name>)  [unwired: 5 in]
            n250 = case shown="真" w430 {
              tunnel: w429 -> [_ w434]
              tunnel: w424 -> [_ w436]
              tunnel: w423 -> [_ w435]
              tunnel: w428 -> [_ w433]
              tunnel: w427 -> [_ w432]
              frame False {
              }
              frame True {
                n251 = global write "CODcr全局变量.vi" "VISA Resource"(w434) -> ()
                n252 = global write "CODcr全局变量.vi" "PORT"(w432) -> ()
                n253 = global write "CODcr全局变量.vi" "IP"(w433) -> ()
                n254 = Bundle By Name(cluster=cluster{"命令":string} {"命令"=""} ("元素"), "命令"="启用模块" ("名称（未命名）")) -> (w437:cluster{"命令":string})
                n255 = Enqueue Element(queue=w436, element=w437, error in (no error)=w435) -> ()  [unwired: 1 in, 3 out]
              }
            }
          }
          frame #1 {
            n256 = call "配置文件保存.vi"() -> ()  [unwired: 12 in]
          }
        }
      }
      event "释放串口": Value Change {
        n257 = event-data() -> ()  [unwired: 1 in, 6 out]
        n258 = Two Button Dialog(message="确认是否释放串口，释放串口将导致通信失败！" ("消息")) -> (T button?=w442:bool)  [unwired: 2 in]
        n259 = case shown="真" w442 {
          tunnel: w441 -> [_ w445]
          tunnel: w440 -> [_ w444]
          frame False {
          }
          frame True {
            n260 = Bundle By Name(cluster=cluster{"命令":string} {"命令"=""} ("元素"), "命令"="停用模块" ("名称（未命名）")) -> (w446:cluster{"命令":string})
            n261 = Enqueue Element(queue=w445, element=w446, error in (no error)=w444) -> ()  [unwired: 1 in, 3 out]
          }
        }
      }
      event "MB通信方式选择": Value Change {
        n262 = event-data() -> ()  [unwired: 1 in, 6 out]
        n263 = flat-sequence {
          frame #0 {
            n264 = global write "CODcr全局变量.vi" "MB通信方式选择"("MB通信方式选择") -> ()
          }
          frame #1 {
            n265 = call "配置文件保存.vi"() -> ()  [unwired: 12 in]
          }
        }
      }
      event "写入消解温度时长": Value Change {
        n266 = event-data() -> ()  [unwired: 1 in, 6 out]
        n267 = local read "消解时长"() -> (w454:u16)
        n268 = local read "消解温度"() -> (w455:u16)
        n269 = Build Array(w455, w454) -> (w453:u16[])
        n270 = call "WordToHex.vi"("WORD"=w453) -> ("数组"=w450:u16[])  [unwired: 10 in]
        n271 = call "CODCrMB_api.vi"("STEP"=enum16{"open", "read", "write", "close"}."write", "values"=w450, "starting address"=u16 4257) -> ()  [unwired: 6 in, 3 out]
      }
      event "校时": Value Change {
        n272 = event-data() -> ()  [unwired: 1 in, 6 out]
        n273 = Get Date/Time In Seconds() -> (seconds since 1Jan1904=w463:timestamp)
        n274 = Build Array(w463) -> (w460:timestamp[])
        n275 = call "DateToHex.vi"("DATE"=w460) -> ("数组"=w459:u16[])  [unwired: 10 in]
        n276 = Insert Into Array(array=u16[] [13] ("values"), index=1 ("索引"), new element=w459) -> (w456:u16[])
        n277 = call "CODCrMB_api.vi"("STEP"=enum16{"open", "read", "write", "close"}."write", "values"=w456, "starting address"=u16 4608) -> ()  [unwired: 6 in, 3 out]
      }
      event "设置": Value Change {
        n278 = event-data() -> ()  [unwired: 1 in, 6 out]
        n279 = property on="窗格" class="Pane"("Origin"=T6 {"Horizontal"=0, "Vertical"=728} ("原点")) -> ()  [unwired: 2 in, 2 out]
        n280 = Bundle By Name(cluster=cluster{"命令":string} {"命令"=""} ("元素"), "命令"="CODCr读取参数" ("名称（未命名）")) -> (w466:cluster{"命令":string})
        n281 = Enqueue Element(queue=w465, element=w466, error in (no error)=w464) -> ()  [unwired: 1 in, 3 out]
      }
      event "返回": Value Change {
        w470 = FALSE ("可见")
        n282 = event-data() -> ()  [unwired: 1 in, 6 out]
        n283 = property on="窗格" class="Pane"("Origin"=T6 {"Horizontal"=0, "Vertical"=0} ("原点")) -> ()  [unwired: 2 in, 2 out]
        n284 = property on="写入消解温度时长" class="Bool"("Visible"=w470) -> ()  [unwired: 2 in, 2 out]
        n285 = property on="释放串口" class="Bool"("Visible"=w470) -> ()  [unwired: 2 in, 2 out]
        n286 = property on="打开串口" class="Bool"("Visible"=w470) -> ()  [unwired: 2 in, 2 out]
        n287 = property on="MB通信方式选择" class="Enum (严格)"("Visible"=w470) -> ()  [unwired: 2 in, 2 out]
      }
      event "曲线斜率K", "曲线截距B", "消解温度", "消解时长": Mouse Down {
        n288 = event-data() -> ("CtlRef"=w474:refnum<vi>)  [unwired: 1 in, 7 out]
        n289 = property class="DigNum"(reference=w474) -> (reference out=w475:refnum<vi>, "Value"=w473:variant)  [unwired: 1 in, 1 out]
        n290 = Variant To Data(Variant=w473) -> (data=w472:sgl)  [unwired: 2 in, 1 out]
        n291 = call "CODCR数字键盘.vi"("OldNumber"=w472) -> ("NewNumber"=w476:sgl)
        n292 = property class="DigNum"(reference=w475, "Value"=w476) -> ()  [unwired: 1 in, 2 out]
      }
      event "隐藏按钮": Value Change {
        n293 = event-data() -> ("NewVal"=w477:bool)  [unwired: 1 in, 5 out]
        n294 = property on="写入消解温度时长" class="Bool"("Visible"=w477) -> ()  [unwired: 2 in, 2 out]
        n295 = property on="释放串口" class="Bool"("Visible"=w477) -> ()  [unwired: 2 in, 2 out]
        n296 = property on="打开串口" class="Bool"("Visible"=w477) -> ()  [unwired: 2 in, 2 out]
        n297 = property on="MB通信方式选择" class="Enum (严格)"("Visible"=w477) -> ()  [unwired: 2 in, 2 out]
      }
    }
  }
  n298 = while {
    tunnel: w6 -> [w479]
    tunnel: w5 -> [w478]
    i -> [w487]
    stop <- FALSE stop-if-true
    n299 = First Call?() -> (First Call?: T/F=w482:bool)
    n300 = case shown="真" w482 {
      tunnel: w479 -> [w491 w496]
      tunnel: w478 -> [w490 w495]
      tunnel: [w491 w494] -> w481
      tunnel: [w490 w493] -> w480
      frame False {
      }
      frame True {
        n301 = Bundle By Name(cluster=cluster{"命令":string} {"命令"=""} ("元素"), "命令"="CODMn读取参数" ("名称（未命名）")) -> (w499:cluster{"命令":string})
        n302 = Enqueue Element(queue=w496, element=w499, timeout in ms (-1)=1000 ("超时毫秒(-1)"), error in (no error)=w495) -> (queue out=w494:refnum<queue>, error out=w493:errorcluster)  [unwired: 1 out]
      }
    }
    n303 = Get Queue Status(queue=w481, error in (no error)=w480) -> (queue out=w485:refnum<queue>, error out=w484:errorcluster, # elements in queue=w486:i32)  [unwired: 1 in, 5 out]
    n304 = Equal To 0?(x=w486) -> (x = 0?=w483:bool)
    n305 = case shown="真" w483 {
      tunnel: w485 -> [_ w501]
      tunnel: w484 -> [_ w500]
      frame False {
      }
      frame True {
        n306 = Bundle By Name(cluster=cluster{"命令":string} {"命令"=""} ("元素"), "命令"="CODCr读取" ("名称（未命名）")) -> (w503:cluster{"命令":string})
        n307 = Enqueue Element(queue=w501, element=w503, timeout in ms (-1)=1000 ("超时毫秒(-1)"), error in (no error)=w500) -> ()  [unwired: 3 out]
      }
    }
    n308 = Wait (ms)(milliseconds to wait=u32 1000 ("等待时间（毫秒）")) -> ()  [unwired: 1 out]
    "主循环次数" <- w487
  }
